vi "queryErrors.vi"(8 "error in (no error)":errorcluster, 11 "VISA resource name":refnum<visa-resource-name>) -> (0 "error out":errorcluster, 2 "Error Register":string, 3 "VISA resource name out":refnum<visa-resource-name>)   [LabVIEW 2023, in "Tti-Pl303Qmd.lvlib"]
doc: "Query all Errors"
uses:
  Tti-Pl303Qmd.lvlib
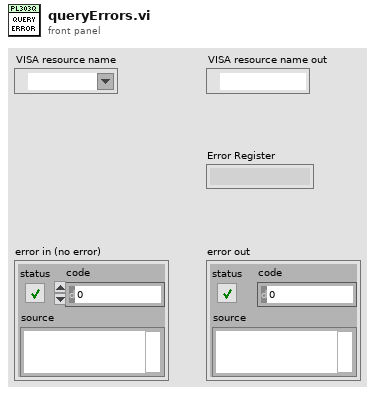
[diagram p1: front panel]
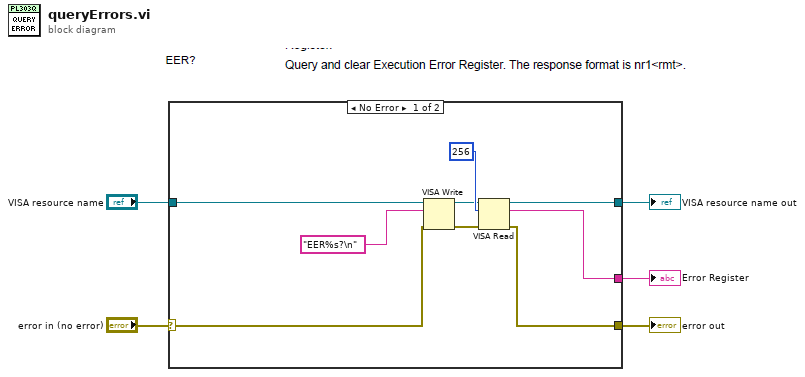
[diagram p0: block diagram]
diagram:
  n1 = case shown="No Error" "error in (no error)" {
    selector: "error in (no error)" -> [w7 w16]
    tunnel: "VISA resource name" -> [w14 w15]
    tunnel: [w9 w16] -> w2
    tunnel: [w11 w15] -> w3
    tunnel: [w8 _] -> w1
    frame No Error {
      n2 = VISA Write(VISA resource name=w14, write buffer="EER%s?\n", error in (no error)=w7) -> (VISA resource name out=w10:refnum<visa-resource-name>, error out=w13:errorcluster)  [unwired: 1 out]
      n3 = VISA Read(VISA resource name=w10, byte count=u32 256, error in (no error)=w13) -> (VISA resource name out=w11:refnum<visa-resource-name>, read buffer=w8:string, error out=w9:errorcluster)  [unwired: 1 out]
    }
    frame Error {
    }
  }
  "error out" <- w2
  "VISA resource name out" <- w3
  "Error Register" <- w1
